vi "PhotonPoseEstimator_Update_All.vi"(9 "Has Results":bool, 10 "PipelineResult":T1={"Targets"=[], "PhotonMultiTargetPNPResult"={"PhotonPNPResult"={"IsPresent"=FALSE, "bestReprojErr"=0.0, "altReprojErr"=0.0, "ambiguity"=0.0, "Best"={"TRANSLATION3D"={"X"=0.0, "Y"=0.0, "Z"=0.0}, "ROTATION3D"={"Q_quaternion"={"R"=1.0, "V"=[0.0, 0.0, 0.0]}}, "XF"=FALSE}, "Alt"={"TRANSLATION3D"={"X"=0.0, "Y"=0.0, "Z"=0.0}, "ROTATION3D"={"Q_quaternion"={"R"=1.0, "V"=[0.0, 0.0, 0.0]}}, "XF"=FALSE}}, "FiducialIDsUsed"=[]}, "PhotonPipelineMetadata"={"CaptureTimestampMicros"=0, "PublishTimestampMicros"=0, "SequenceID"=0, "TimeSinceLastPong"=0}} {"PhotonMultiTargetPNPResult"."PhotonPNPResult"."Alt"."TRANSLATION3D"."Z" format="%14.3f"; "PhotonMultiTargetPNPResult"."PhotonPNPResult"."Alt"."TRANSLATION3D"."Y" format="%14.3f"; "PhotonMultiTargetPNPResult"."PhotonPNPResult"."Alt"."TRANSLATION3D"."X" format="%14.3f"; "PhotonMultiTargetPNPResult"."PhotonPNPResult"."Best"."TRANSLATION3D"."Z" format="%14.3f"; "PhotonMultiTargetPNPResult"."PhotonPNPResult"."Best"."TRANSLATION3D"."Y" format="%14.3f"; "PhotonMultiTargetPNPResult"."PhotonPNPResult"."Best"."TRANSLATION3D"."X" format="%14.3f"; "Targets"."AltCameraToTarget"."TRANSLATION3D"."Z" format="%14.3f"; "Targets"."AltCameraToTarget"."TRANSLATION3D"."Y" format="%14.3f"; "Targets"."AltCameraToTarget"."TRANSLATION3D"."X" format="%14.3f"; "Targets"."BestCameraToTarget"."TRANSLATION3D"."Z" format="%14.3f"; "Targets"."BestCameraToTarget"."TRANSLATION3D"."Y" format="%14.3f"; "Targets"."BestCameraToTarget"."TRANSLATION3D"."X" format="%14.3f"}, 11 "PhotonPoseEstimator":T14={"LastPose"={"Translation3d"={"X"=0.0, "Y"=0.0, "Z"=0.0}, "Rotation3d"={"Q_quaternion"={"R"=1.0, "V"=[0.0, 0.0, 0.0]}}}, "ReferencePose"={"Translation3d"={"X"=0.0, "Y"=0.0, "Z"=0.0}, "Rotation3d"={"Q_quaternion"={"R"=1.0, "V"=[0.0, 0.0, 0.0]}}}, "FieldTags"={"AprilTagMap"={}, "FieldLength"=0.0, "FieldWidth"=0.0, "OriginPosition "=enum."kBlueAllianceWallRightSide,", "OriginPose3d"={"Translation3d"={"X"=0.0, "Y"=0.0, "Z"=0.0}, "Rotation3d"={"Q_quaternion"={"R"=1.0, "V"=[0.0, 0.0, 0.0]}}}}, "PrimaryStratety"=enum."LOWEST_AMBIGUITY", "Camera"="", "RobotToCamera"={"TRANSLATION3D"={"X"=0.0, "Y"=0.0, "Z"=0.0}, "ROTATION3D"={"Q_quaternion"={"R"=1.0, "V"=[0.0, 0.0, 0.0]}}, "XF"=FALSE}, "ReportedErrors"=[], "HighestAmbiguity"=10.0, "MultiTagFallbackStrategy"=enum."LOWEST_AMBIGUITY", "PoseCacheTimeoutSec"=-1.0, "PhotonTargetModel"={"Vertices"=[], "IsPlaner"=FALSE, "IsSpherical"=FALSE}, "BaseNTName"="/photonvision"} {"PhotonTargetModel"."Vertices"."Z" format="%14.3f"; "PhotonTargetModel"."Vertices"."Y" format="%14.3f"; "PhotonTargetModel"."Vertices"."X" format="%14.3f"; "RobotToCamera"."TRANSLATION3D"."Z" format="%14.3f"; "RobotToCamera"."TRANSLATION3D"."Y" format="%14.3f"; "RobotToCamera"."TRANSLATION3D"."X" format="%14.3f"; "FieldTags"."OriginPose3d"."Translation3d"."Z" format="%14.3f"; "FieldTags"."OriginPose3d"."Translation3d"."Y" format="%14.3f"; "FieldTags"."OriginPose3d"."Translation3d"."X" format="%14.3f"; "ReferencePose"."Translation3d"."Z" format="%14.3f"; "ReferencePose"."Translation3d"."Y" format="%14.3f"; "ReferencePose"."Translation3d"."X" format="%14.3f"; "LastPose"."Translation3d"."Z" format="%14.3f"; "LastPose"."Translation3d"."Y" format="%14.3f"; "LastPose"."Translation3d"."X" format="%14.3f"}) -> (1 "Pos Found":bool, 2 "PhotonEstimatedRobotPose":T11={"EstimatedPose"={"Translation3d"={"X"=0.0, "Y"=0.0, "Z"=0.0}, "Rotation3d"={"Q_quaternion"={"R"=1.0, "V"=[0.0, 0.0, 0.0]}}}, "TimeStamp_Seconds"=0.0, "targetsUsed"=[], "Strategy"=enum."LOWEST_AMBIGUITY"} {"targetsUsed"."AltCameraToTarget"."TRANSLATION3D"."Z" format="%14.3f"; "targetsUsed"."AltCameraToTarget"."TRANSLATION3D"."Y" format="%14.3f"; "targetsUsed"."AltCameraToTarget"."TRANSLATION3D"."X" format="%14.3f"; "targetsUsed"."BestCameraToTarget"."TRANSLATION3D"."Z" format="%14.3f"; "targetsUsed"."BestCameraToTarget"."TRANSLATION3D"."Y" format="%14.3f"; "targetsUsed"."BestCameraToTarget"."TRANSLATION3D"."X" format="%14.3f"; "EstimatedPose"."Translation3d"."Z" format="%14.3f"; "EstimatedPose"."Translation3d"."Y" format="%14.3f"; "EstimatedPose"."Translation3d"."X" format="%14.3f"}, 3 "out PhotonPoseEstimator":T14={"LastPose"={"Translation3d"={"X"=0.0, "Y"=0.0, "Z"=0.0}, "Rotation3d"={"Q_quaternion"={"R"=1.0, "V"=[0.0, 0.0, 0.0]}}}, "ReferencePose"={"Translation3d"={"X"=0.0, "Y"=0.0, "Z"=0.0}, "Rotation3d"={"Q_quaternion"={"R"=1.0, "V"=[0.0, 0.0, 0.0]}}}, "FieldTags"={"AprilTagMap"={}, "FieldLength"=0.0, "FieldWidth"=0.0, "OriginPosition "=enum."kBlueAllianceWallRightSide,", "OriginPose3d"={"Translation3d"={"X"=0.0, "Y"=0.0, "Z"=0.0}, "Rotation3d"={"Q_quaternion"={"R"=1.0, "V"=[0.0, 0.0, 0.0]}}}}, "PrimaryStratety"=enum."LOWEST_AMBIGUITY", "Camera"="", "RobotToCamera"={"TRANSLATION3D"={"X"=0.0, "Y"=0.0, "Z"=0.0}, "ROTATION3D"={"Q_quaternion"={"R"=1.0, "V"=[0.0, 0.0, 0.0]}}, "XF"=FALSE}, "ReportedErrors"=[], "HighestAmbiguity"=10.0, "MultiTagFallbackStrategy"=enum."LOWEST_AMBIGUITY", "PoseCacheTimeoutSec"=-1.0, "PhotonTargetModel"={"Vertices"=[], "IsPlaner"=FALSE, "IsSpherical"=FALSE}, "BaseNTName"="/photonvision"} {"PhotonTargetModel"."Vertices"."Z" format="%14.3f"; "PhotonTargetModel"."Vertices"."Y" format="%14.3f"; "PhotonTargetModel"."Vertices"."X" format="%14.3f"; "RobotToCamera"."TRANSLATION3D"."Z" format="%14.3f"; "RobotToCamera"."TRANSLATION3D"."Y" format="%14.3f"; "RobotToCamera"."TRANSLATION3D"."X" format="%14.3f"; "FieldTags"."OriginPose3d"."Translation3d"."Z" format="%14.3f"; "FieldTags"."OriginPose3d"."Translation3d"."Y" format="%14.3f"; "FieldTags"."OriginPose3d"."Translation3d"."X" format="%14.3f"; "ReferencePose"."Translation3d"."Z" format="%14.3f"; "ReferencePose"."Translation3d"."Y" format="%14.3f"; "ReferencePose"."Translation3d"."X" format="%14.3f"; "LastPose"."Translation3d"."Z" format="%14.3f"; "LastPose"."Translation3d"."Y" format="%14.3f"; "LastPose"."Translation3d"."X" format="%14.3f"})   [LabVIEW 2019, in "PhotonVisionLib.lvlib"]
doc: "Provided data from polling a camera, updates the estimated position of the robot. Returns empty if:\n - New data has not been received since the last call to update.\n - No targets were found from the camera\n - There is no camera set\n\n\nInputs:\n -- PhotonPoseEstimator -- data cluster -- Data guiding how the position determination is done.\n -- PipelineResults -- data cluster -- Data provided from PhotonCamera_GetLatestResults.\n -- HasResults -- boolean - TRUE if targets have been identified in the Pipeline results. This can be provided by PhotonCamera_GetLatestResults.\n -- cameraMatrix -- matrix -- Camera calibration data that can be used in the case of no assigned PhotonCamera.\n -- distCoeffs -- matrix -- Camera calibration data that can be used in the case of no assigned PhotonCamera\n\nOutputs:\n -- PhotonPoseEstimator -- data cluster -- Updated data cluster.\n -- PhotonEstimatedRobotPose -- data cluster -- Estimated robot position, timestamp, and targets used to create the estimte.\n -- PosFound -- boolean -- A position has been determined."
uses:
  PhotonVisionLib.lvlib
  <vilib>/Rock Robotics/WPI/ThirdParty/JAS_Junk/TrajLib/TypeDef/TRANSLATION3D.ctl
  <vilib>/Rock Robotics/WPI/ThirdParty/JAS_Junk/TrajLib/Trajectory_Library.lvlib
  <vilib>/Rock Robotics/WPI/ThirdParty/JAS_Junk/TrajLib/TypeDef/QUATERNION.ctl
  <vilib>/Rock Robotics/WPI/ThirdParty/JAS_Junk/TrajLib/TypeDef/ROTATION3D.ctl
  <vilib>/Rock Robotics/WPI/ThirdParty/JAS_Junk/TrajLib/TypeDef/POSE3D.ctl
  TypeDef/PhotonEstimatedRobotPoseType.ctl
  Enum/PhotonPoseStrategy_ENUM.ctl
  TypeDef/TargetCornerType.ctl
  <vilib>/Rock Robotics/WPI/ThirdParty/JAS_Junk/TrajLib/TypeDef/TRANSFORM3D.ctl
  TypeDef/PhotonTrackedTargetType.ctl
  <vilib>/Rock Robotics/WPI/ThirdParty/JAS_Junk/TrajLib/TypeDef/AprilTag.ctl
  <vilib>/Rock Robotics/WPI/ThirdParty/JAS_Junk/TrajLib/Enum/AprilTagFieldLayoutOrignPosition_ENUM.ctl
  <vilib>/Rock Robotics/WPI/ThirdParty/JAS_Junk/TrajLib/TypeDef/AprilTagFieldLayout.ctl
  TypeDef/PhotonPoseEstimatorType.ctl
  TypeDef/PhotonPipelineResultType.ctl
  TypeDef/PhotonPNPResultType.ctl
  TypeDef/PhotonMultiTargetPNPResultType.ctl
  TypeDef/PhotonTargetModel.ctl
  TypeDef/PhotonPipelineMetadataType.ctl
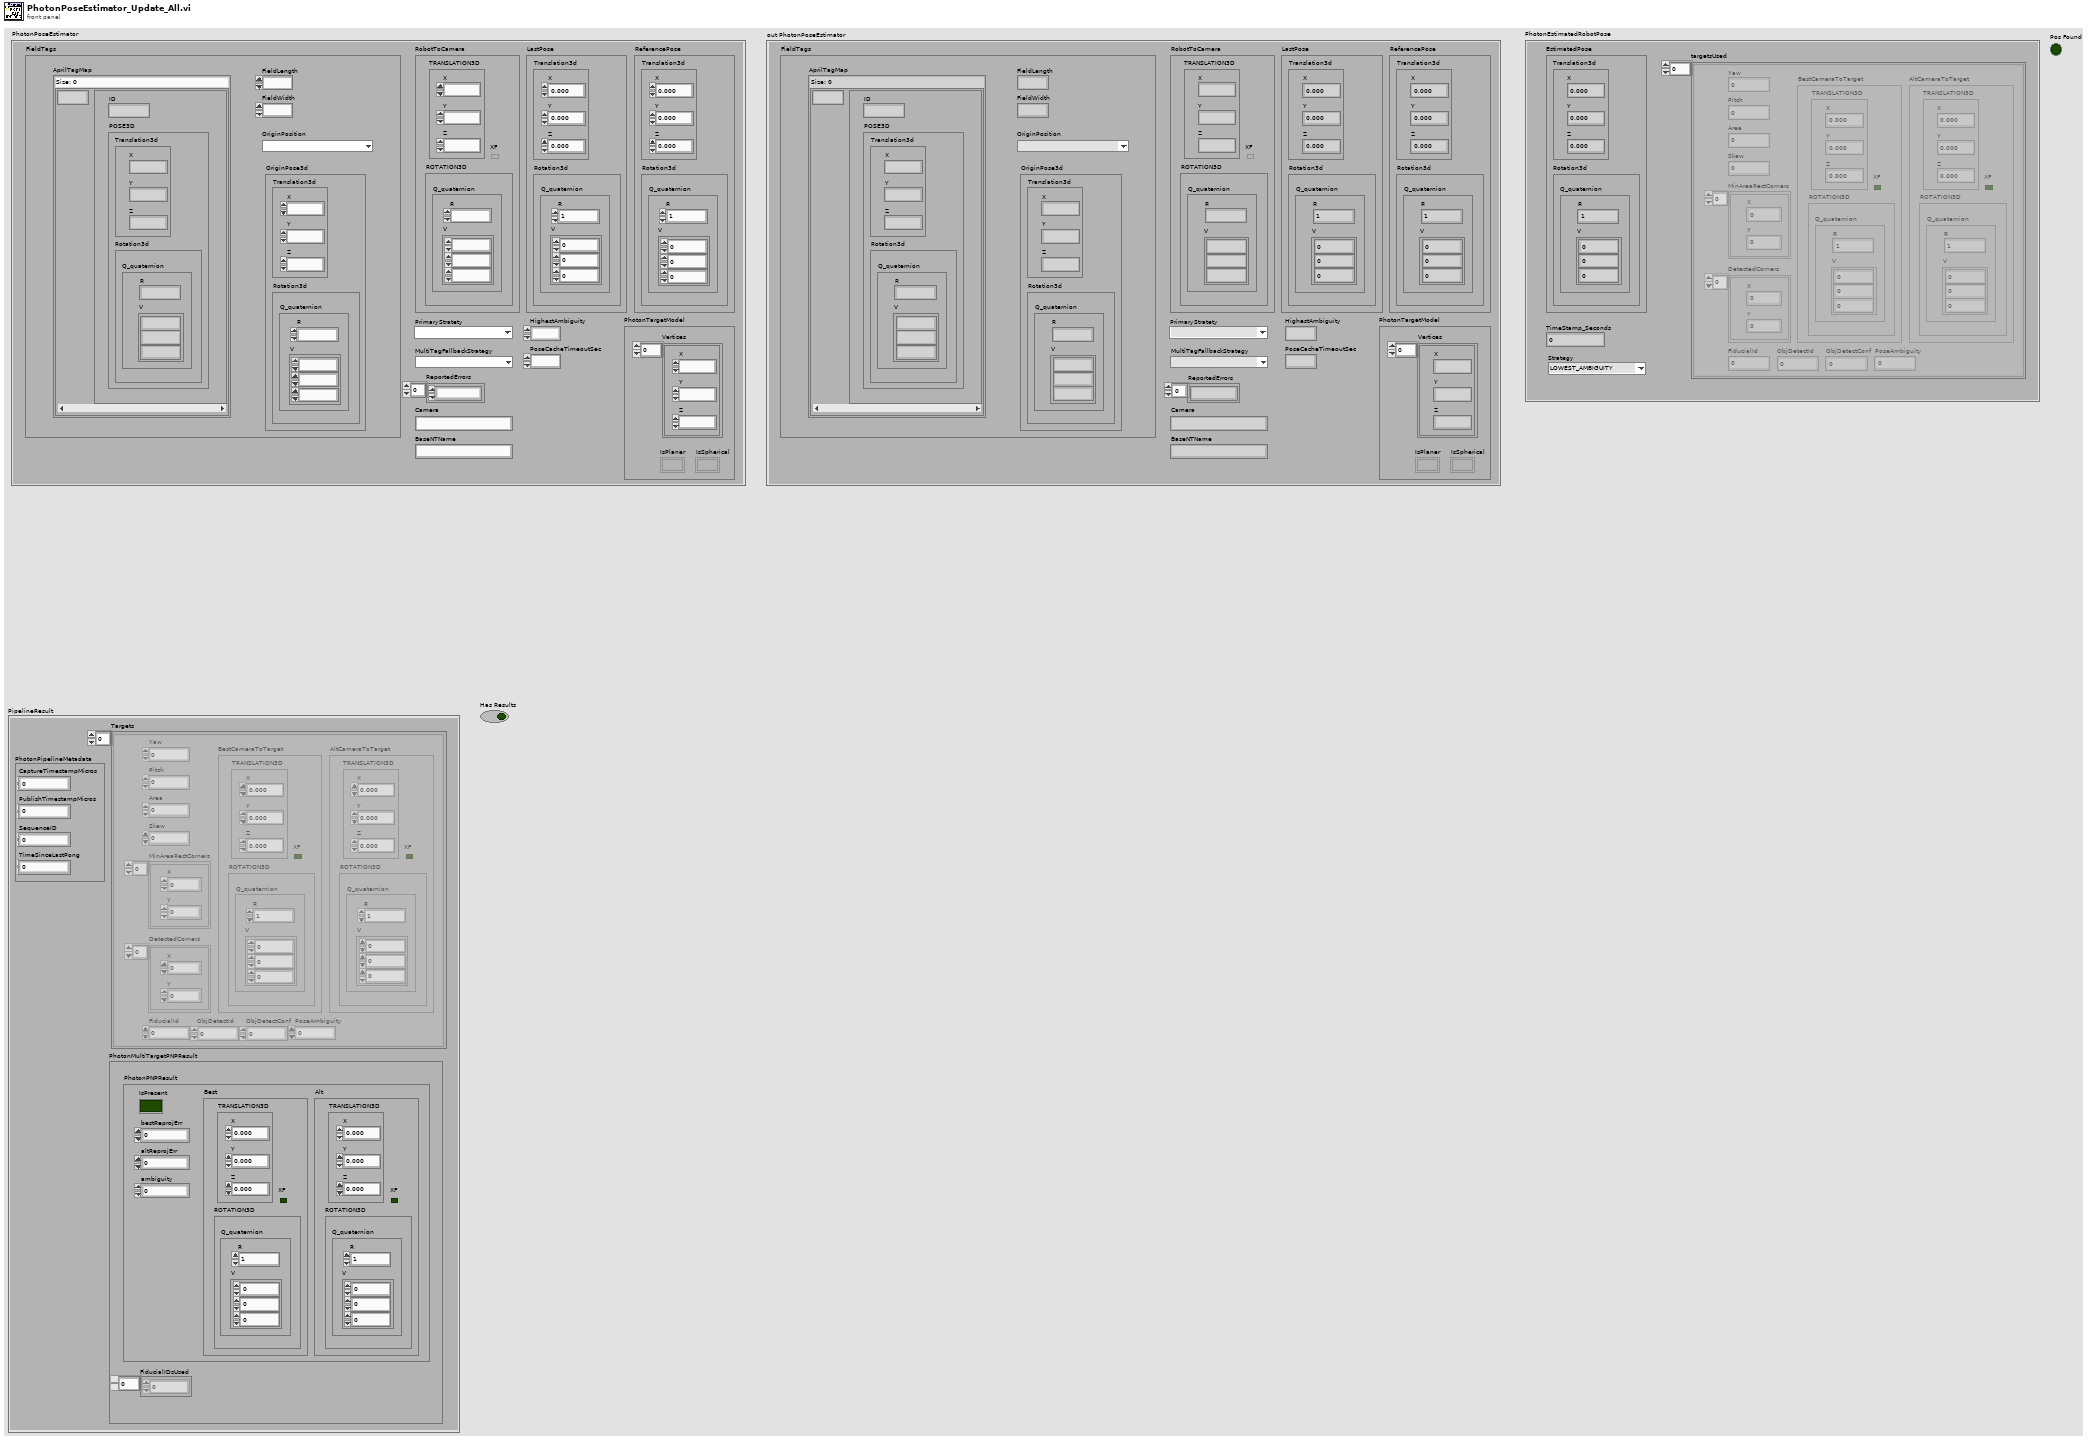
[diagram p1: front panel]
types:
  T1 = typedef "PhotonVisionLib.lvlib/PhotonPipelineResultType.ctl" = cluster{"Targets":T2[], "PhotonMultiTargetPNPResult":T8, "PhotonPipelineMetadata":T10}
  T2 = typedef "PhotonVisionLib.lvlib/PhotonTrackedTargetType.ctl" = cluster{"Yaw":dbl, "Pitch":dbl, "Area":dbl, "Skew":dbl, "MinAreaRectCorners":T3[], "BestCameraToTarget":T4, "FiducialId":i32, "AltCameraToTarget":T4, "PoseAmbiguity":dbl, "DetectedCorners":T3[], "ObjDetectId":i32, "ObjDetectConf":sgl}
  T3 = typedef "PhotonVisionLib.lvlib/TargetCornerType.ctl" = cluster{"X":dbl, "Y":dbl}
  T4 = typedef "Trajectory_Library.lvlib/TRANSFORM3D.ctl" = cluster{"TRANSLATION3D":T5, "ROTATION3D":T6, "XF":bool}
  T5 = typedef "Trajectory_Library.lvlib/TRANSLATION3D.ctl" = cluster{"X":dbl, "Y":dbl, "Z":dbl}
  T6 = typedef "Trajectory_Library.lvlib/ROTATION3D.ctl" = cluster{"Q_quaternion":T7}
  T7 = typedef "Trajectory_Library.lvlib/QUATERNION.ctl" = cluster{"R":dbl, "V":dbl[]}
  T8 = typedef "PhotonVisionLib.lvlib/PhotonMultiTargetPNPResultType.ctl" = cluster{"PhotonPNPResult":T9, "FiducialIDsUsed":i16[]}
  T9 = typedef "PhotonVisionLib.lvlib/PhotonPNPResultType.ctl" = cluster{"IsPresent":bool, "bestReprojErr":dbl, "altReprojErr":dbl, "ambiguity":dbl, "Best":T4, "Alt":T4}
  T10 = typedef "PhotonVisionLib.lvlib/PhotonPipelineMetadataType.ctl" = cluster{"CaptureTimestampMicros":i64, "PublishTimestampMicros":i64, "SequenceID":i64, "TimeSinceLastPong":i64}
  T11 = typedef "PhotonVisionLib.lvlib/PhotonEstimatedRobotPoseType.ctl" = cluster{"EstimatedPose":T12, "TimeStamp_Seconds":dbl, "targetsUsed":T2[], "Strategy":T13}
  T12 = typedef "Trajectory_Library.lvlib/POSE3D.ctl" = cluster{"Translation3d":T5, "Rotation3d":T6}
  T13 = typedef "PhotonVisionLib.lvlib/PhotonPoseStrategy_ENUM.ctl" = enum16{"LOWEST_AMBIGUITY", "CLOSEST_TO_CAMERA_HEIGHT", "CLOSEST_TO_REFERENCE_POSE", "CLOSEST_TO_LAST_POSE", "AVERAGE_BEST_TARGETS", "MULTI_TAG_PNP_ON_COPROCESSOR", "MULTI_TAG_PNP_ON_RIO", "PNP_DISTANCE_TRIG_SOLVE", "CONSTRAINED_SOLVEPNP"}
  T14 = typedef "PhotonVisionLib.lvlib/PhotonPoseEstimatorType.ctl" = cluster{"LastPose":T12, "ReferencePose":T12, "FieldTags":T15, "PrimaryStratety":T13, "Camera":string, "RobotToCamera":T4, "ReportedErrors":dbl[], "HighestAmbiguity":dbl, "MultiTagFallbackStrategy":T13, "PoseCacheTimeoutSec":dbl, "PhotonTargetModel":T18, "BaseNTName":string}
  T15 = typedef "Trajectory_Library.lvlib/AprilTagFieldLayout.ctl" = cluster{"AprilTagMap":map{i32, T16}, "FieldLength":dbl, "FieldWidth":dbl, "OriginPosition ":T17, "OriginPose3d":T12}
  T16 = typedef "Trajectory_Library.lvlib/AprilTag.ctl" = cluster{"ID":i32, "POSE3D":T12}
  T17 = typedef "Trajectory_Library.lvlib/AprilTagFieldLayoutOrignPosition_ENUM.ctl" = enum16{"kBlueAllianceWallRightSide,", "kRedAllianceWallRightSide,"}
  T18 = typedef "PhotonVisionLib.lvlib/PhotonTargetModel.ctl" = cluster{"Vertices":T5[], "IsPlaner":bool, "IsSpherical":bool}
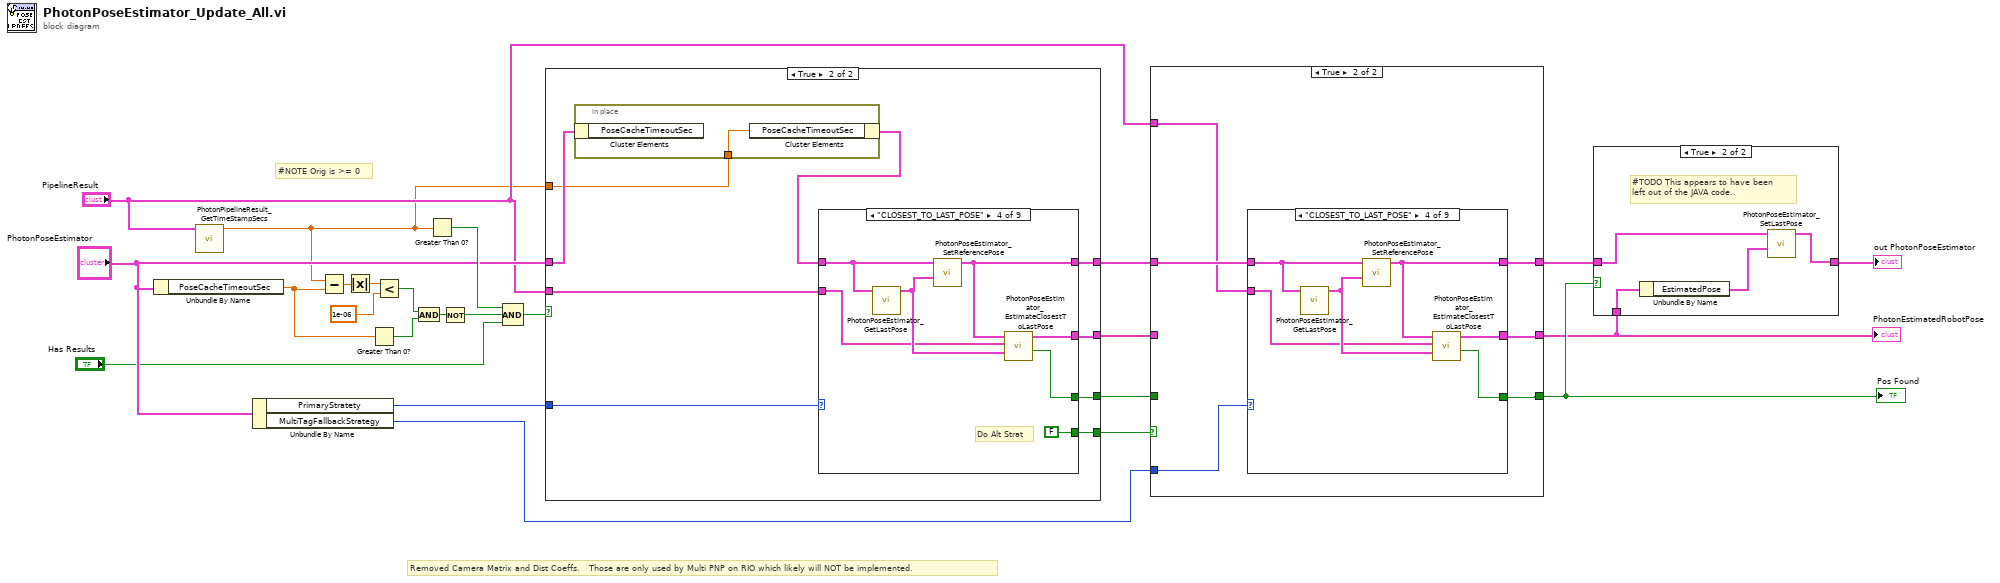
[diagram p0: block diagram]
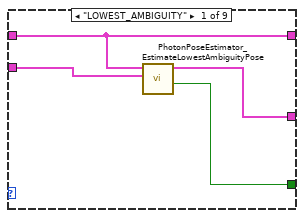
[diagram p3: hidden frame]
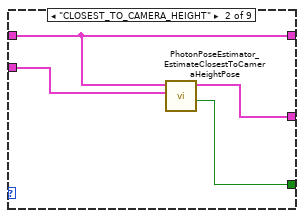
[diagram p4: hidden frame]
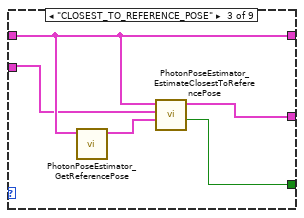
[diagram p5: hidden frame]
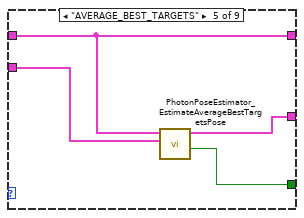
[diagram p6: hidden frame]
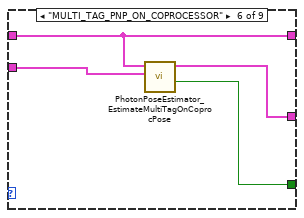
[diagram p7: hidden frame]
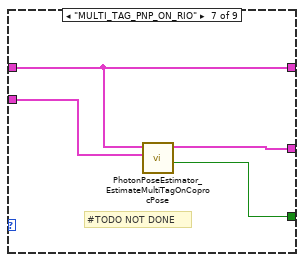
[diagram p8: hidden frame]
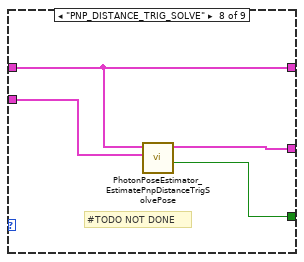
[diagram p9: hidden frame]
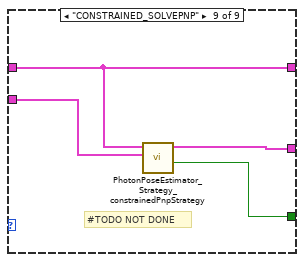
[diagram p10: hidden frame]
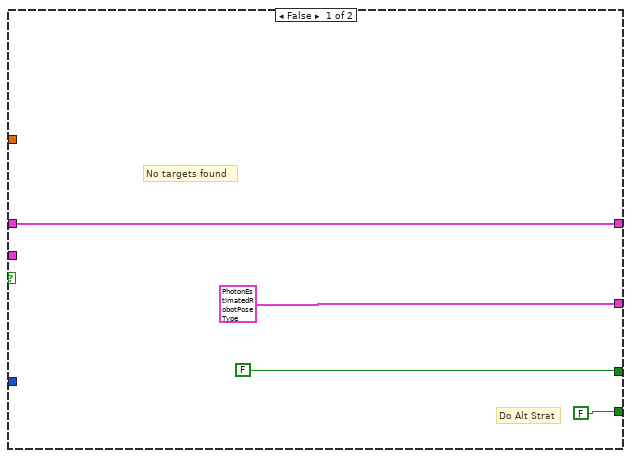
[diagram p11: hidden frame]
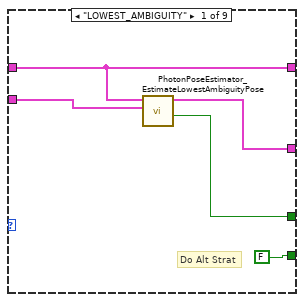
[diagram p12: hidden frame]
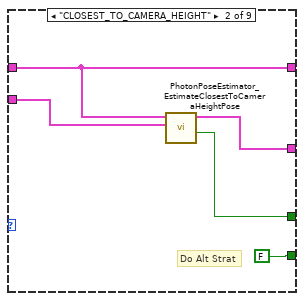
[diagram p13: hidden frame]
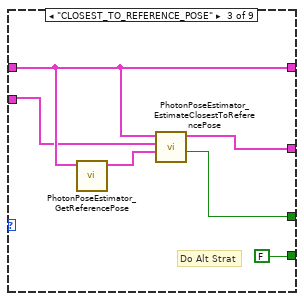
[diagram p14: hidden frame]
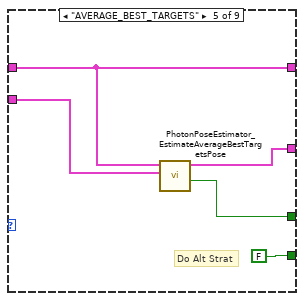
[diagram p15: hidden frame]
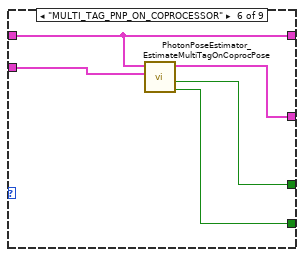
[diagram p16: hidden frame]
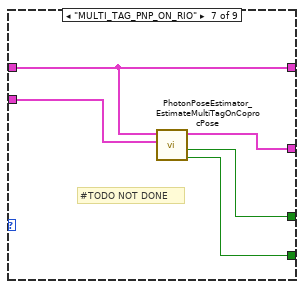
[diagram p17: hidden frame]
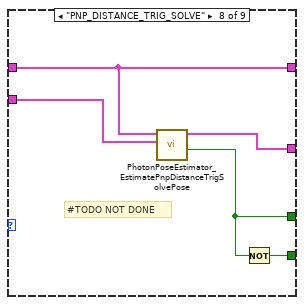
[diagram p18: hidden frame]
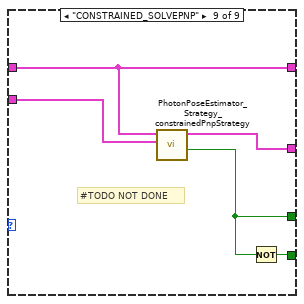
[diagram p19: hidden frame]
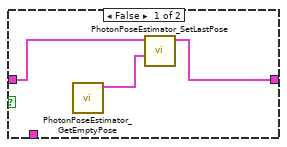
[diagram p20: hidden frame]
diagram:
  # "Removed Camera Matrix and Dist Coeffs.   Those are only used by Multi PNP on RIO which likely will NOT be implemented."
  # "#NOTE Orig is >= 0"
  n1 = Unbundle By Name("PhotonPoseEstimator") -> ("PoseCacheTimeoutSec"=w18:dbl)
  n2 = call "PhotonPipelineResult_GetTimeStampSecs.vi"("PhotonPipelineResult"="PipelineResult") -> ("TimeStampSec"=w1:dbl)  [unwired: 10 in]
  n3 = Unbundle By Name("PhotonPoseEstimator") -> ("PrimaryStratety"=w24:T13, "MultiTagFallbackStrategy"=w3:T13)
  n4 = Subtract(x=w1, y=w18) -> (x-y=w17:dbl)
  n5 = Absolute Value(x=w17) -> (abs(x)=w16:dbl)
  n6 = Greater Than 0?(x=w18) -> (x > 0?=w13:bool)
  n7 = Less?(x=w16, y=1e-06) -> (x < y?=w14:bool)
  n8 = And(x=w14, y=w13) -> (x .and. y?=w12:bool)
  n9 = Greater Than 0?(x=w1) -> (x > 0?=w21:bool)
  n10 = Not(x=w12) -> (.not. x?=w11:bool)
  n11 = Compound Arithmetic op=AND(w21, w11, "Has Results") -> (w22:bool)
  n12 = case shown="True" w22 {
    tunnel: [w28 w35] -> w5
    tunnel: "PhotonPoseEstimator" -> [w28 w32]
    tunnel: [T11 {"EstimatedPose"={"Translation3d"={"X"=0.0, "Y"=0.0, "Z"=0.0}, "Rotation3d"={"Q_quaternion"={"R"=1.0, "V"=[0.0, 0.0, 0.0]}}}, "TimeStamp_Seconds"=0.0, "targetsUsed"=[], "Strategy"=enum."LOWEST_AMBIGUITY"} ("PhotonEstimatedRobotPose") w33] -> w7
    tunnel: [FALSE w34] -> w9
    tunnel: w24 -> [_ w37]
    tunnel: "PipelineResult" -> [_ w36]
    tunnel: w1 -> [_ w30]
    tunnel: [FALSE ("Do Alt Strategy") w29] -> w10
    frame False {
      # "Do Alt Strat"
      # "No targets found"
    }
    frame True {
      n13 = in-place {
        in-place-border: w30 -> [w38]
        n14 = in-place-cluster #1(w32) -> ()  [unwired: 1 out]
        n15 = in-place-cluster #1("PoseCacheTimeoutSec"=w38) -> (w31:T14)
      }
      n16 = case shown="\"CLOSEST_TO_LAST_POSE\"" w37 {
        tunnel: w36 -> [w40 w45 w50 w57 w63 w70 w75 w80 w85]
        tunnel: w31 -> [w41 w46 w51 w61 w64 w71 w76 w81 w86]
        tunnel: [w41 w46 w51 w56 w64 w71 w76 w81 w86] -> w35
        tunnel: [w43 w47 w52 w58 w65 w68 w73 w77 w82] -> w34
        tunnel: [w42 w48 w53 w59 w66 w69 w74 w79 w84] -> w33
        tunnel: [FALSE ("Do Alt Strategy") FALSE ("Do Alt Strategy") FALSE ("Do Alt Strategy") FALSE ("Do Alt Strategy") FALSE ("Do Alt Strategy") w67 w72 w78 w83] -> w29
        frame "LOWEST_AMBIGUITY" {
          # "Do Alt Strat"
          n17 = call "PhotonPoseEstimator_EstimateLowestAmbiguityPose.vi"("CameraResult"=w40, "PhotoPoseEstimator"=w41) -> ("Pos Found"=w43:bool, "PhotonEstimatedRobotPose"=w42:T11)  [unwired: 8 in]
        }
        frame "CLOSEST_TO_CAMERA_HEIGHT" {
          # "Do Alt Strat"
          n18 = call "PhotonPoseEstimator_EstimateClosestToCameraHeightPose.vi"("CameraResult"=w45, "PhotoPoseEstimator"=w46) -> ("Pos Found"=w47:bool, "PhotonEstimatedRobotPose"=w48:T11)  [unwired: 8 in]
        }
        frame "CLOSEST_TO_REFERENCE_POSE" {
          # "Do Alt Strat"
          n19 = call "PhotonPoseEstimator_GetReferencePose.vi"("PhotonPoseEstimator"=w51) -> ("ReferencePose"=w54:T12)  [unwired: 10 in]
          n20 = call "PhotonPoseEstimator_EstimateClosestToReferencePose.vi"("ReferencePose"=w54, "CameraResult"=w50, "PhotoPoseEstimator"=w51) -> ("Pos Found"=w52:bool, "PhotonEstimatedRobotPose"=w53:T11)  [unwired: 7 in]
        }
        frame "CLOSEST_TO_LAST_POSE" {
          # "Do Alt Strat"
          n21 = call "PhotonPoseEstimator_GetLastPose.vi"("PhotonPoseEstimator"=w61) -> ("LastPose"=w60:T12)  [unwired: 10 in]
          n22 = call "PhotonPoseEstimator_SetReferencePose.vi"("ReferencePose"=w60, "PhotonPoseEstimator"=w61) -> ("out PhotonPoseEstimator"=w56:T14)  [unwired: 9 in]
          n23 = call "PhotonPoseEstimator_EstimateClosestToLastPose.vi"("LastPose"=w60, "CameraResult"=w57, "PhotoPoseEstimator"=w56) -> ("Pos Found"=w58:bool, "PhotonEstimatedRobotPose"=w59:T11)  [unwired: 7 in]
        }
        frame "AVERAGE_BEST_TARGETS" {
          # "Do Alt Strat"
          n24 = call "PhotonPoseEstimator_EstimateAverageBestTargetsPose.vi"("CameraResult"=w63, "PhotoPoseEstimator"=w64) -> ("Pos Found"=w65:bool, "PhotonEstimatedRobotPose"=w66:T11)  [unwired: 8 in]
        }
        frame "MULTI_TAG_PNP_ON_COPROCESSOR" {
          n25 = call "PhotonPoseEstimator_EstimateMultiTagOnCoprocPose.vi"("CameraResult"=w70, "PhotoPoseEstimator"=w71) -> ("Do Alt Strategy"=w67:bool, "Pos Found"=w68:bool, "PhotonEstimatedRobotPose"=w69:T11)  [unwired: 7 in]
        }
        frame "MULTI_TAG_PNP_ON_RIO" {
          # "#TODO NOT DONE"
          n26 = call "PhotonPoseEstimator_EstimateMultiTagOnCoprocPose.vi"("CameraResult"=w75, "PhotoPoseEstimator"=w76) -> ("Do Alt Strategy"=w72:bool, "Pos Found"=w73:bool, "PhotonEstimatedRobotPose"=w74:T11)  [unwired: 7 in]
        }
        frame "PNP_DISTANCE_TRIG_SOLVE" {
          # "#TODO NOT DONE"
          n27 = call "PhotonPoseEstimator_EstimatePnpDistanceTrigSolvePose.vi"("CameraResult"=w80, "PhotoPoseEstimator"=w81) -> ("Pos Found"=w77:bool, "PhotonEstimatedRobotPose"=w79:T11)  [unwired: 8 in]
          n28 = Not(x=w77) -> (.not. x?=w78:bool)
        }
        frame "CONSTRAINED_SOLVEPNP" {
          # "#TODO NOT DONE"
          n29 = call "PhotonPoseEstimator_Strategy_constrainedPnpStrategy.vi"("CameraResult"=w85, "PhotoPoseEstimator"=w86) -> ("Pos Found"=w82:bool, "PhotonEstimatedRobotPose"=w84:T11)  [unwired: 8 in]
          n30 = Not(x=w82) -> (.not. x?=w83:bool)
        }
      }
    }
  }
  n31 = case shown="True" w10 {
    tunnel: [w89 w90] -> w8
    tunnel: w9 -> [w89 _]
    tunnel: w7 -> [w88 _]
    tunnel: [w88 w91] -> w6
    tunnel: w5 -> [w87 w95]
    tunnel: [w87 w92] -> w4
    tunnel: "PipelineResult" -> [_ w94]
    tunnel: w3 -> [_ w93]
    frame False {
    }
    frame True {
      n32 = case shown="\"CLOSEST_TO_LAST_POSE\"" w93 {
        tunnel: w94 -> [w96 w100 w104 w110 w115 w121 w123 w127 w131]
        tunnel: w95 -> [w97 w101 w105 w114 w116 w122 w124 w128 w132]
        tunnel: [w97 w101 w105 w109 w116 w122 w124 w128 w132] -> w92
        tunnel: [w99 w102 w106 w111 w117 w119 w125 w129 w133] -> w90
        tunnel: [w98 w103 w107 w112 w118 w120 w126 w130 w134] -> w91
        frame "LOWEST_AMBIGUITY" {
          n33 = call "PhotonPoseEstimator_EstimateLowestAmbiguityPose.vi"("CameraResult"=w96, "PhotoPoseEstimator"=w97) -> ("Pos Found"=w99:bool, "PhotonEstimatedRobotPose"=w98:T11)  [unwired: 8 in]
        }
        frame "CLOSEST_TO_CAMERA_HEIGHT" {
          n34 = call "PhotonPoseEstimator_EstimateClosestToCameraHeightPose.vi"("CameraResult"=w100, "PhotoPoseEstimator"=w101) -> ("Pos Found"=w102:bool, "PhotonEstimatedRobotPose"=w103:T11)  [unwired: 8 in]
        }
        frame "CLOSEST_TO_REFERENCE_POSE" {
          n35 = call "PhotonPoseEstimator_GetReferencePose.vi"("PhotonPoseEstimator"=w105) -> ("ReferencePose"=w108:T12)  [unwired: 10 in]
          n36 = call "PhotonPoseEstimator_EstimateClosestToReferencePose.vi"("ReferencePose"=w108, "CameraResult"=w104, "PhotoPoseEstimator"=w105) -> ("Pos Found"=w106:bool, "PhotonEstimatedRobotPose"=w107:T11)  [unwired: 7 in]
        }
        frame "CLOSEST_TO_LAST_POSE" {
          n37 = call "PhotonPoseEstimator_GetLastPose.vi"("PhotonPoseEstimator"=w114) -> ("LastPose"=w113:T12)  [unwired: 10 in]
          n38 = call "PhotonPoseEstimator_SetReferencePose.vi"("ReferencePose"=w113, "PhotonPoseEstimator"=w114) -> ("out PhotonPoseEstimator"=w109:T14)  [unwired: 9 in]
          n39 = call "PhotonPoseEstimator_EstimateClosestToLastPose.vi"("LastPose"=w113, "CameraResult"=w110, "PhotoPoseEstimator"=w109) -> ("Pos Found"=w111:bool, "PhotonEstimatedRobotPose"=w112:T11)  [unwired: 7 in]
        }
        frame "AVERAGE_BEST_TARGETS" {
          n40 = call "PhotonPoseEstimator_EstimateAverageBestTargetsPose.vi"("CameraResult"=w115, "PhotoPoseEstimator"=w116) -> ("Pos Found"=w117:bool, "PhotonEstimatedRobotPose"=w118:T11)  [unwired: 8 in]
        }
        frame "MULTI_TAG_PNP_ON_COPROCESSOR" {
          n41 = call "PhotonPoseEstimator_EstimateMultiTagOnCoprocPose.vi"("CameraResult"=w121, "PhotoPoseEstimator"=w122) -> ("Pos Found"=w119:bool, "PhotonEstimatedRobotPose"=w120:T11)  [unwired: 7 in, 1 out]
        }
        frame "MULTI_TAG_PNP_ON_RIO" {
          # "#TODO NOT DONE"
          n42 = call "PhotonPoseEstimator_EstimateMultiTagOnCoprocPose.vi"("CameraResult"=w123, "PhotoPoseEstimator"=w124) -> ("Pos Found"=w125:bool, "PhotonEstimatedRobotPose"=w126:T11)  [unwired: 7 in, 1 out]
        }
        frame "PNP_DISTANCE_TRIG_SOLVE" {
          # "#TODO NOT DONE"
          n43 = call "PhotonPoseEstimator_EstimatePnpDistanceTrigSolvePose.vi"("CameraResult"=w127, "PhotoPoseEstimator"=w128) -> ("Pos Found"=w129:bool, "PhotonEstimatedRobotPose"=w130:T11)  [unwired: 8 in]
        }
        frame "CONSTRAINED_SOLVEPNP" {
          # "#TODO NOT DONE"
          n44 = call "PhotonPoseEstimator_Strategy_constrainedPnpStrategy.vi"("CameraResult"=w131, "PhotoPoseEstimator"=w132) -> ("Pos Found"=w133:bool, "PhotonEstimatedRobotPose"=w134:T11)  [unwired: 8 in]
        }
      }
    }
  }
  "PhotonEstimatedRobotPose" <- w6
  "Pos Found" <- w8
  n45 = case shown="True" w8 {
    tunnel: w4 -> [w136 w141]
    tunnel: [w137 w140] -> w23
    tunnel: w6 -> [_ w139]
    frame False {
      n46 = call "PhotonPoseEstimator_GetEmptyPose.vi"() -> ("EmptyPose"=w135:T12)  [unwired: 11 in]
      n47 = call "PhotonPoseEstimator_SetLastPose.vi"("LastPose"=w135, "PhotonPoseEstimator"=w136) -> ("out PhotonPoseEstimator"=w137:T14)  [unwired: 9 in]
    }
    frame True {
      # "#TODO This appears to have been\nleft out of the JAVA code.."
      n48 = Unbundle By Name(w139) -> ("EstimatedPose"=w138:T12)
      n49 = call "PhotonPoseEstimator_SetLastPose.vi"("LastPose"=w138, "PhotonPoseEstimator"=w141) -> ("out PhotonPoseEstimator"=w140:T14)  [unwired: 9 in]
    }
  }
  "out PhotonPoseEstimator" <- w23
